vi "Compute Dialog Position.vi"(6 "graph pane width":u32, 7 "offset":T1={"Left"=-638, "Top"=81}, 9 "launch button position":T1, 10 "launch button bounds":T3, 11 "front panel bounds":T2) -> (3 "variant with position attribute":variant)   [LabVIEW 2024, in "Dynamic Signal Acquisition (Interactive) UI.lvlib"]
uses:
  Dynamic Signal Acquisition (Interactive) UI.lvlib
  <vilib>/Utility/miscctls.llb/LVPositionTypeDef.ctl
  <vilib>/Utility/miscctls.llb/LVBoundsTypeDef.ctl
  <vilib>/Utility/miscctls.llb/LVRectTypeDef.ctl
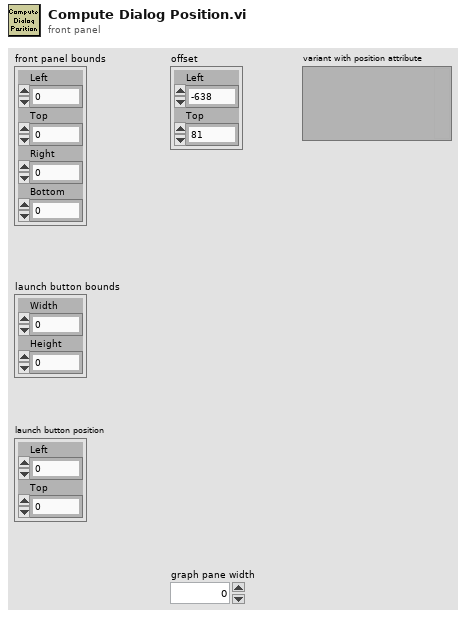
[diagram p1: front panel]
types:
  T1 = typedef "LVPositionTypeDef.ctl" = cluster{"Left":i32, "Top":i32}
  T2 = typedef "LVRectTypeDef.ctl" = cluster{"Left":i16, "Top":i16, "Right":i16, "Bottom":i16}
  T3 = typedef "LVBoundsTypeDef.ctl" = cluster{"Width":u32, "Height":u32}
  T4 = cluster{"Left":i32, "Top":i32, "Right":i32, "Bottom":i32}
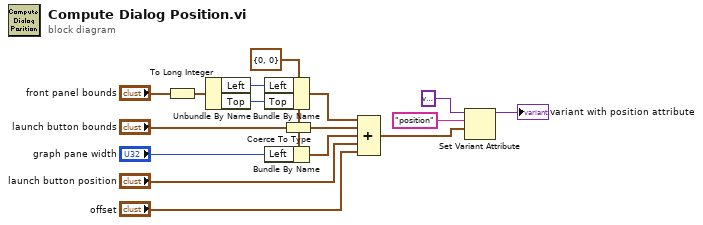
[diagram p0: block diagram]
diagram:
  w16 = T1 {"Left"=0, "Top"=0} ("Position")
  n1 = To Long Integer(number="front panel bounds") -> (32bit integer=w3:T4)
  n2 = Unbundle By Name(w3) -> ("Left"=w11:i32, "Top"=w12:i32)
  n3 = Bundle By Name(cluster=w16, "Left"=w11, "Top"=w12) -> (w13:T1)
  n4 = Bundle By Name(cluster=w16, "Left"="graph pane width") -> (w9:T1)
  n5 = Coerce To Type(0:"launch button bounds", 1:w16) -> (2:w15:T1)
  n6 = Compound Arithmetic op=ADD(w13, w15, w9, "launch button position", "offset") -> (w5:T1)
  n7 = Set Variant Attribute(Variant=variant ("variant"), name="position" ("f"), value=w5) -> (Variant out=→"variant with position attribute":variant)  [unwired: 1 in, 2 out]
